vi "PRACTICA 5 DIVISOR DE VOLTAJE.vi"() -> ()   [LabVIEW 2017]
panel:
  in  "?":dbl
  in  "?":dbl
  in  "?":dbl
  in  "?":dbl
  in  "?":dbl
  out "POTENCIA R2":dbl
  out "POTENCIA R3":dbl
  out "CORRIENTE R3":dbl
  out "CORRIENTE R2":dbl
  out "POTENCIA R1":dbl
  out "VOLTAJE R3 2":dbl
  out "CORRIENTE R1":dbl
  out "VOLTAJE R2":dbl
  out "?":dbl
  out "CORRIENTE VF2":dbl
  out "CORRIENTE VF1":dbl
  # "PRACTICA 5"
  # "MODELADO DE CIRCUITO ELECTRICO."
  # "VOLTAJE R1"
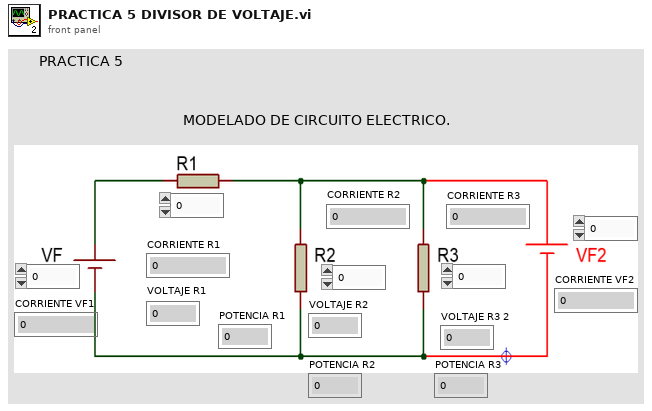
[diagram p1: front panel]
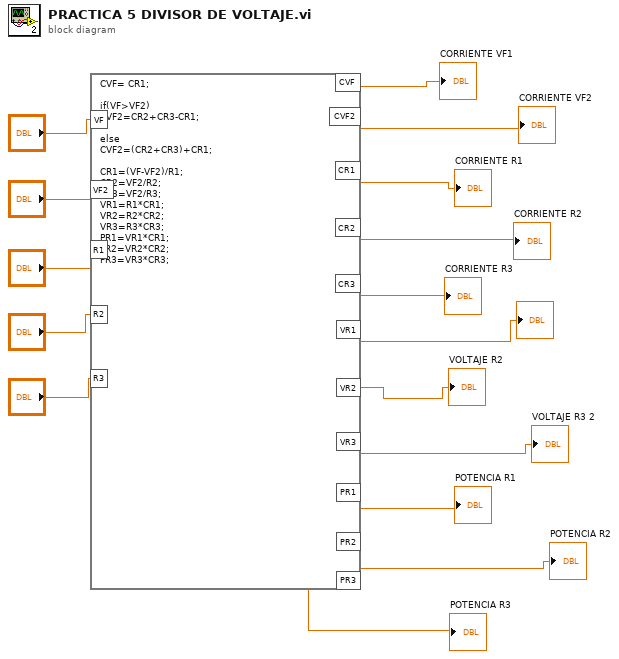
[diagram p0: block diagram]
diagram:
  n1 = formula code="CVF= CR1;\n\nif(VF>VF2)\nCVF2=CR2+CR3-CR1;\n\nelse\nCVF2=(CR2+CR3)+CR1;\n\nCR1=(VF-VF2)/R1;\nCR2=VF2/R2;\nCR3=VF2/R3;\nVR1=R1*CR1;\nVR2=R2*CR2;\nVR3=R3*CR3;\nPR1=VR1*CR1;\nPR2=VR2*CR2;\nPR3=VR3*CR3;"("VF2"="?", "R1"="?", "R2"="?", "R3"="?", "VF"="?") -> ("CR1"=→"CORRIENTE R1":dbl, "CR3"=→"CORRIENTE R3":dbl, "VR1"=→"?":dbl, "VR2"=→"VOLTAJE R2":dbl, "VR3"=→"VOLTAJE R3 2":dbl, "PR1"=→"POTENCIA R1":dbl, "CR2"=→"CORRIENTE R2":dbl, "CVF2"=→"CORRIENTE VF2":dbl, "CVF"=→"CORRIENTE VF1":dbl, "PR2"=→"POTENCIA R2":dbl, "PR3"=→"POTENCIA R3":dbl)
